vi "splitParAndArg.vi"(8 "paraEndMark":string=";", 9 "paraStartMark":string="=", 10 "allArguments":string="CF_Lvr_PButtonStatus,2,0,0,1,CF_Lvr_PButtonStatus_Reversed,1,0,0,1,CF_Lvr_RButtonStatus,2,0,0,1,CF_Lvr_RButtonStatus_Reversed,1,0,0,1,CF_Lvr_NButtonStatus,2,0,0,1,CF_Lvr_NButtonStatus_Reversed,1,0,0,1,CF_Lvr_DButtonStatus,2,0,0,1,CF_Lvr_DButtonStatus_Reversed,1,0,0,1,CF_Lvr_PRelStat,2,0,0,1,CF_Lvr_PRelButStatus_Reversed,1,0,0,1", 11 "allParameters":string="productPwmInMode = char signame[],float updateSigVal_i,int msWaitBefCheck,int demandRes_k_i,int demandRes_b") -> (1 "argArray":string[](array[string])=["CF_Lvr_PButtonStatus", "2", "0", "0", "1", "CF_Lvr_PButtonStatus_Reversed", "1", "0", "0", "1", "CF_Lvr_RButtonStatus", "2", "0", "0", "1", "CF_Lvr_RButtonStatus_Reversed", "1", "0", "0", "1", "CF_Lvr_NButtonStatus", "2", "0", "0", "1", "CF_Lvr_NButtonStatus_Reversed", "1", "0", "0", "1", "CF_Lvr_DButtonStatus", "2", "0", "0", "1", "CF_Lvr_DButtonStatus_Reversed", "1", "0", "0", "1", "CF_Lvr_PRelStat", "2", "0", "0", "1", "CF_Lvr_PRelButStatus_Reversed", "1", "0", "0", "1"], 2 "paraArray":string[](array[string])=["char signame[]", "float updateSigVal_i", "int msWaitBefCheck", "int demandRes_k_i", "int demandRes_b"], 3 "sameNum?":bool)   [LabVIEW 2010]
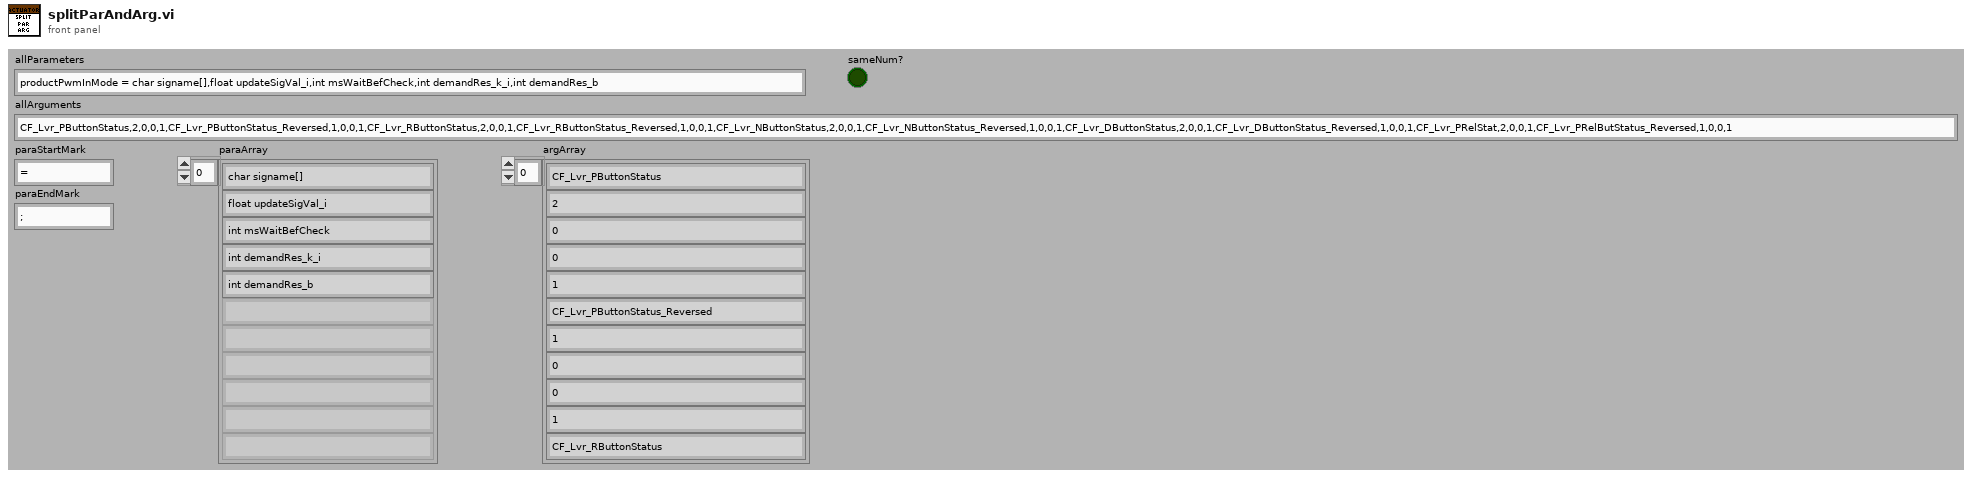
[diagram p1: front panel]
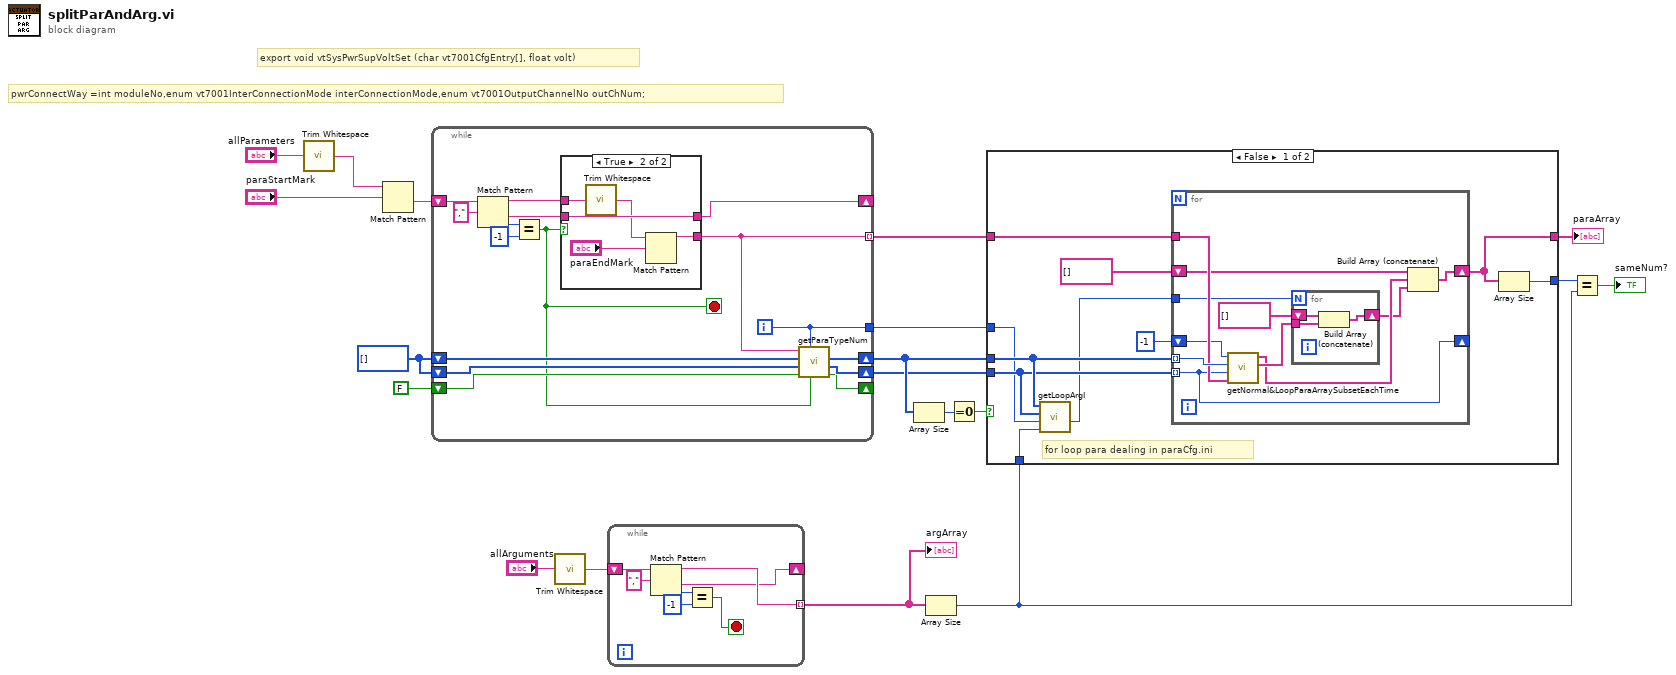
[diagram p0: block diagram]
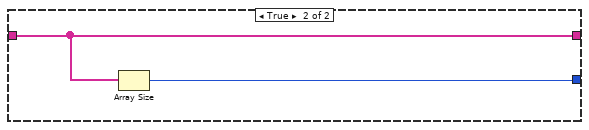
[diagram p2: hidden frame]
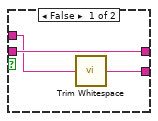
[diagram p3: hidden frame]
diagram:
  w11 = i32[] []
  # "pwrConnectWay =int moduleNo,enum vt7001InterConnectionMode interConnectionMode,enum vt7001OutputChannelNo outChNum;"
  # "export void vtSysPwrSupVoltSet (char vt7001CfgEntry[], float volt)"
  n1 = call <vilib>:"Trim Whitespace.vi"("string"="allParameters") -> ("trimmed string"=w15:string)  [unwired: 1 in]
  n2 = Match Pattern(string=w15, regular expression="paraStartMark") -> (after substring=w19:string)  [unwired: 1 in, 3 out]
  n3 = while {
    shift-right: [w29] -> _
    shift-left: w19 -> [w35]
    tunnel: [w21] -> w7 mode=indexing
    shift-right: [w27] -> w4
    shift-left: w11 -> [w28]
    shift-right: [w25] -> w3
    shift-left: w11 -> [w26]
    shift-right: [w23] -> _
    shift-left: FALSE ("lastTimeLoopParaExist?") -> [w24]
    tunnel: [w20] -> w1
    i -> [w20]
    stop <- w22 stop-if-true
    n4 = Match Pattern(string=w35, regular expression=",") -> (before substring=w31:string, after substring=w30:string, offset past match=w33:i32)  [unwired: 1 in, 1 out]
    n5 = Equal?(x=w33, y=-1) -> (x = y?=w22:bool)
    n6 = case shown="True" w22 {
      tunnel: w31 -> [w37 w40]
      tunnel: [w36 w43] -> w21
      tunnel: w30 -> [w38 w42]
      tunnel: [w38 w42] -> w29
      frame False {
        n7 = call <vilib>:"Trim Whitespace.vi"("string"=w37) -> ("trimmed string"=w36:string)  [unwired: 1 in]
      }
      frame True {
        n8 = call <vilib>:"Trim Whitespace.vi"("string"=w40) -> ("trimmed string"=w39:string)  [unwired: 1 in]
        n9 = Match Pattern(string=w39, regular expression="paraEndMark") -> (before substring=w43:string)  [unwired: 1 in, 3 out]
      }
    }
    n10 = call "getParaTypeNum.vi"("testEnd"=w22, "paraSN"=w20, "lastTimeLoopParaExist?"=w24, "lastTimeLoopParaEndNumArr"=w26, "lastTimeLoopParaStartNumArr"=w28, "parameter"=w21) -> ("thisTimeLoopParaExist?"=w23:bool, "thisTimeLoopParaEndNumArr"=w25:i32[], "thisTimeLoopParaStartNumArr"=w27:i32[])  [unwired: 3 in]
  }
  n11 = call <vilib>:"Trim Whitespace.vi"("string"="allArguments") -> ("trimmed string"=w13:string)  [unwired: 1 in]
  n12 = while {
    shift-right: [w45] -> _
    shift-left: w13 -> [w50]
    tunnel: [w46] -> w18 mode=indexing
    stop <- w44 stop-if-true
    n13 = Match Pattern(string=w50, regular expression=",") -> (before substring=w46:string, after substring=w45:string, offset past match=w48:i32)  [unwired: 1 in, 1 out]
    n14 = Equal?(x=w48, y=-1) -> (x = y?=w44:bool)
  }
  "argArray" <- w18
  n15 = Array Size(array=w4) -> (size(s)=w8:i32)
  n16 = Array Size(array=w18) -> (size(s)=w2:i32)
  n17 = Equal To 0?(x=w8) -> (x = 0?=w9:bool)
  n18 = case shown="False" w9 {
    tunnel: w7 -> [w60 w76]
    tunnel: [w52 w76] -> w6
    tunnel: [w53 w75] -> w5
    tunnel: w4 -> [w58 _]
    tunnel: w3 -> [w57 _]
    tunnel: w2 -> [w51 _]
    tunnel: w1 -> [w56 _]
    frame False {
      # "for loop para dealing in paraCfg.ini"
      n19 = call "getLoopArgI.vi"("argNum"=w51, "paraNum"=w56, "loopParaEndNumArr"=w57, "loopParaStartNumArr"=w58) -> ("loopArgI"=w55:i32)  [unwired: 5 in, 2 out]
      n20 = for {
        tunnel: w58 -> [w71] mode=indexing
        tunnel: w57 -> [w68] mode=indexing
        tunnel: w60 -> [w70]
        shift-right: [w68] -> _
        shift-left: -1 -> [w69]
        shift-right: [w63] -> w52
        shift-left: string[] [] -> [w67]
        tunnel: w55 -> [w65]
        n21 = call "getNormal&LoopParaArraySubsetEachTime.vi"("paraArray"=w70, "loopParaEndNum"=w68, "loopParaStartNum"=w71, "lastLoopParaEndNum"=w69) -> ("loopParaArray"=w66:string[], "normalParaArray"=w62:string[])  [unwired: 6 in]
        n22 = for {
          N: w65 -> [_]
          tunnel: w66 -> [w73]
          shift-right: [w72] -> w61
          shift-left: string[] [] -> [w74]
          n23 = Build Array (concatenate)(w74, w73) -> (w72:string[])
        }
        n24 = Build Array (concatenate)(w67, w62, w61) -> (w63:string[])
      }
      n25 = Array Size(array=w52) -> (size(s)=w53:i32)
    }
    frame True {
      n26 = Array Size(array=w76) -> (size(s)=w75:i32)
    }
  }
  "paraArray" <- w6
  n27 = Equal?(x=w5, y=w2) -> (x = y?=→"sameNum?":bool)
